vi "Sample-2.vi"() -> ()   [LabVIEW 2016]
uses:
  <vilib>/NI/Modbus Library/API/Wrapper/Create TCP Master.vi
  <vilib>/NI/Modbus Library/API/Wrapper/API Main.lvlib
panel:
  in  "Boolean 3":bool
  in  "stop":bool
  out "Tab Control":T1(tab)
  out "Boolean":bool
  out "SB-01-B-IAC 12":dbl
  out "SB-01-B-VAC 12":dbl
  out "SB-01-B-IAC 11":dbl
  out "SB-01-B-VAC 11":dbl
  out "SB-01-A-IAC 8":dbl
  out "SB-01-A-VAC 8":dbl
  out "SB-01-B-IAC 10":dbl
  out "SB-01-B-VAC 10":dbl
  out "SB-01-A-IAC 7":dbl
  out "SB-01-A-VAC 7":dbl
  out "SB-01-PAC 4":dbl
  out "SB-01-B-IAC 9":dbl
  out "SB-01-B-VAC 9":dbl
  out "SB-01-B-IAC 8":dbl
  out "SB-01-B-VAC 8":dbl
  out "SB-01-A-IAC 6":dbl
  out "SB-01-A-VAC 6":dbl
  out "SB-01-B-IAC 7":dbl
  out "SB-01-B-VAC 7":dbl
  out "SB-01-A-IAC 5":dbl
  out "SB-01-A-VAC 5":dbl
  out "SB-01-PAC 3":dbl
  out "SB-01-B-IAC 6":dbl
  out "SB-01-B-VAC 6":dbl
  out "SB-01-B-IAC 5":dbl
  out "SB-01-B-VAC 5":dbl
  out "SB-01-A-IAC 4":dbl
  out "SB-01-A-VAC 4":dbl
  out "SB-01-B-IAC 4":dbl
  out "SB-01-B-VAC 4":dbl
  out "SB-01-A-IAC 3":dbl
  out "SB-01-A-VAC 3":dbl
  out "SB-01-PAC 2":dbl
  out "SB-01-B-IAC 3":dbl
  out "SB-01-B-VAC 3":dbl
  out "SB-01-B-IAC 2":dbl
  out "SB-01-B-VAC 2":dbl
  out "SB-01-A-IAC 2":dbl
  out "SB-01-A-VAC 2":dbl
  out "SB-01-B-IAC":dbl
  out "SB-01-B-VAC":dbl
  out "SB-01-A-IAC":dbl
  out "SB-01-A-VAC":dbl
  out "SB-01-PAC":dbl
  out "PM-01-FREQ 2":dbl
  out "SI-M-FREQ 6":dbl
  out "SI-M-L3 6":dbl
  out "SI-M-L2 6":dbl
  out "SI-M-L1 6":dbl
  out "SI-M-PAC 6":dbl
  out "SI-M-FREQ 5":dbl
  out "SI-M-L3 5":dbl
  out "SI-M-L2 5":dbl
  out "SI-M-L1 5":dbl
  out "SI-M-PAC 5":dbl
  out "SI-M-FREQ 4":dbl
  out "SI-M-L3 4":dbl
  out "SI-M-L2 4":dbl
  out "SI-M-L1 4":dbl
  out "SI-M-PAC 4":dbl
  out "SI-M-FREQ 3":dbl
  out "SI-M-L3 3":dbl
  out "SI-M-L2 3":dbl
  out "SI-M-L1 3":dbl
  out "SI-M-PAC 3":dbl
  out "SI-M-FREQ 2":dbl
  out "SI-M-L3 2":dbl
  out "SI-M-L2 2":dbl
  out "SI-M-L1 2":dbl
  out "SI-M-PAC 2":dbl
  out "SI-M-FREQ":dbl
  out "SI-M-L3":dbl
  out "SI-M-L2":dbl
  out "SI-M-L1":dbl
  out "SI-M-PAC":dbl
  out "BANK-01-TEMP 2":dbl
  out "BANK-01-IDC 2":dbl
  out "BANK-01-VDC 2":dbl
  out "BANK-01-SOC 2":dbl
  out "BANK-01-TEMP":dbl
  out "BANK-01-IDC":dbl
  out "BANK-01-VDC":dbl
  out "BANK-01-SOC":dbl
  out "BANK-01-TEMP 4":dbl
  out "BANK-01-IDC 4":dbl
  out "BANK-01-VDC 4":dbl
  out "BANK-01-SOC 4":dbl
  out "BANK-01-TEMP 3":dbl
  out "BANK-01-IDC 3":dbl
  out "BANK-01-VDC 3":dbl
  out "BANK-01-SOC 3":dbl
  out "PM-01-FREQ":dbl
  out "PM-01-IAC":dbl
  out "PM-01-VAC":dbl
  out "PM-01-PAC":dbl
  out "Boolean 2":bool
  in  "SB-05-IPADDRESS 3":string caption="SB-01-IPADDRESS"
  in  "SB-05-PORT 3":string
  in  "SB-04-PORT 2":string
  in  "SB-04-IPADDRESS 2":string caption="SB-01-IPADDRESS"
  in  "SB-03-PORT 2":string
  in  "SB-03-IPADDRESS 2":string caption="SB-01-IPADDRESS"
  in  "SB-02-PORT 2":string
  in  "SB-02-IPADDRESS 2":string caption="SB-01-IPADDRESS"
  in  "SB-01-PORT 2":string
  in  "SB-01-IPADDRESS 2":string caption="SB-01-IPADDRESS"
  in  "SB-05-IPADDRESS 2":string caption="SB-01-IPADDRESS"
  in  "SB-05-PORT 2":string
  in  "INTERVAL":string(combo)
  in  "setting_save_mysql":bool
  in  "db_pwd":string caption="SB-01-IPADDRESS"
  in  "db_username":string caption="SB-01-IPADDRESS"
  in  "db_database":string caption="SB-01-IPADDRESS"
  in  "db_port":string caption="SB-01-IPADDRESS"
  in  "db_host":string caption="SB-01-IPADDRESS"
  in  "db_connection":string caption="SB-01-IPADDRESS"
  in  "setting_save":bool
  in  "SB-04-PORT":string
  in  "SB-04-IPADDRESS":string caption="SB-01-IPADDRESS"
  in  "SB-03-PORT":string
  in  "SB-03-IPADDRESS":string caption="SB-01-IPADDRESS"
  in  "SB-02-PORT":string
  in  "SB-02-IPADDRESS":string caption="SB-01-IPADDRESS"
  in  "SB-01-PORT":string
  in  "SB-01-IPADDRESS":string
  in  "SB-05-IPADDRESS":string caption="SB-01-IPADDRESS"
  in  "SB-05-PORT":string
  in  "Multicolumn Listbox":i32(listbox)
  in  "Path":path
  in  "DATE_END":timestamp format="%<%d/%m/%Y>T"
  in  "DATE_START":timestamp format="%<%d/%m/%Y>T"
  in  "DOWNLOAD":bool
  out "AC_VOLTAGE":cluster{dbl, dbl}[](graph)
  out "BATTERY_CURRENT":cluster{dbl, dbl}[](graph)
  out "SOC":cluster{dbl, dbl}[](graph)
  out "AC_POWER":cluster{dbl, dbl}[](graph)
  in  "Radio Buttons":T2(radio)
  # "RUMAH BUJAH ( 36.58 kWp )"
  # "STP-01"
  # "C.Vdc(V)"
  # "BANK-1"
  # "BANK-2"
  # "BANK-3"
  # "BANK-4"
  # "Pac (W)"
  # "C.Idc(A)"
  # "SOC (%)"
  # "SOC (%)"
  # "SOC (%)"
  # "SOC (%)"
  # "A.Vdc(V)"
  # "D.Vdc(V)"
  # "V_bat(V)"
  # "V_bat(V)"
  # "V_bat(V)"
  # "V_bat(V)"
  # "A.Idc(A)"
  # "D.Idc(A)"
  # "I_bat(A)"
  # "I_bat(A)"
  # "I_bat(A)"
  # "I_bat(A)"
  # "B.Vdc(V)"
  # "E.Vdc(V)"
  # "T_bat(°C)"
  # "T_bat(°C)"
  # "T_bat(°C)"
  # "T_bat(°C)"
  # "B.Idc(A)"
  # "E.Idc(A)"
  # "SI-M"
  # "SI-M"
  # "SI-01"
  # "SI-02"
  # "SI-01"
  # "SI-02"
  # "Pac (W)"
  # "Pac (W)"
  # "Pac (W)"
  # "Pac (W)"
  # "Pac (W)"
  # "Pac (W)"
  # "L1"
  # "L1"
  # "L1"
  # "L1"
  # "L1"
  # "L1"
  # "L2"
  # "L2"
  # "L2"
  # "L2"
  # "L2"
  # "L2"
  # "L3"
  # "L3"
  # "L3"
  # "L3"
  # "L3"
  # "L3"
  # "Fz(HZ)"
  # "Fz(HZ)"
  # "Fz(HZ)"
  # "Fz(HZ)"
  # "Fz(HZ)"
  # "Fz(HZ)"
  # "PM-01"
  # "Pac(W)"
  # "L1"
  # "L2"
  # "L3"
  # "fz(hz)"
  # "STP-04"
  # "C.Vdc(V)"
  # "Pac (W)"
  # "C.Idc(A)"
  # "A.Vdc(V)"
  # "D.Vdc(V)"
  # "A.Idc(A)"
  # "D.Idc(A)"
  # "B.Vdc(V)"
  # "E.Vdc(V)"
  # "B.Idc(A)"
  # "E.Idc(A)"
  # "STP-03"
  # "C.Vdc(V)"
  # "Pac (W)"
  # "C.Idc(A)"
  # "A.Vdc(V)"
  # "D.Vdc(V)"
  # "A.Idc(A)"
  # "D.Idc(A)"
  # "B.Vdc(V)"
  # "E.Vdc(V)"
  # "B.Idc(A)"
  # "E.Idc(A)"
  # "STP-02"
  # "C.Vdc(V)"
  # "Pac (W)"
  # "C.Idc(A)"
  # "A.Vdc(V)"
  # "D.Vdc(V)"
  # "A.Idc(A)"
  # "D.Idc(A)"
  # "B.Vdc(V)"
  # "E.Vdc(V)"
  # "B.Idc(A)"
  # "E.Idc(A)"
  # "SETTING"
  # "MODBUS TCP IP"
  # "MYSQL DATABASE"
  # "STP-01"
  # "SI-02"
  # "DB_CONNECTION :"
  # "IP ADDRESS"
  # "IP ADDRESS"
  # "DB_HOST :"
  # "PORT"
  # "PORT"
  # "DB_PORT  :"
  # "STP-02"
  # "SI-03"
  # "DB_DATABASE  :"
  # "IP ADDRESS"
  # "IP ADDRESS"
  # "DB_USERNAME  :"
  # "PORT"
  # "PORT"
  # "DB_PASSWORD  :"
  # "INTERVAL  :"
  # "STP-03"
  # "SI-04"
  # "IP ADDRESS"
  # "IP ADDRESS"
  # "PORT"
  # "PORT"
  # "STP-04"
  # "SI-05"
  # "IP ADDRESS"
  # "IP ADDRESS"
  # "PORT"
  # "PORT"
  # "SI-01"
  # "SI-06"
  # "IP ADDRESS"
  # "IP ADDRESS"
  # "PORT"
  # "PORT"
  # "DATA MANAGER"
  # "IP ADDRESS"
  # "PORT"
  # "ALERT LIST"
  # "DOWNLOAD DATA"
  # "FILE"
  # "DATE (START)"
  # "DATE (END)"
  # "CHART"
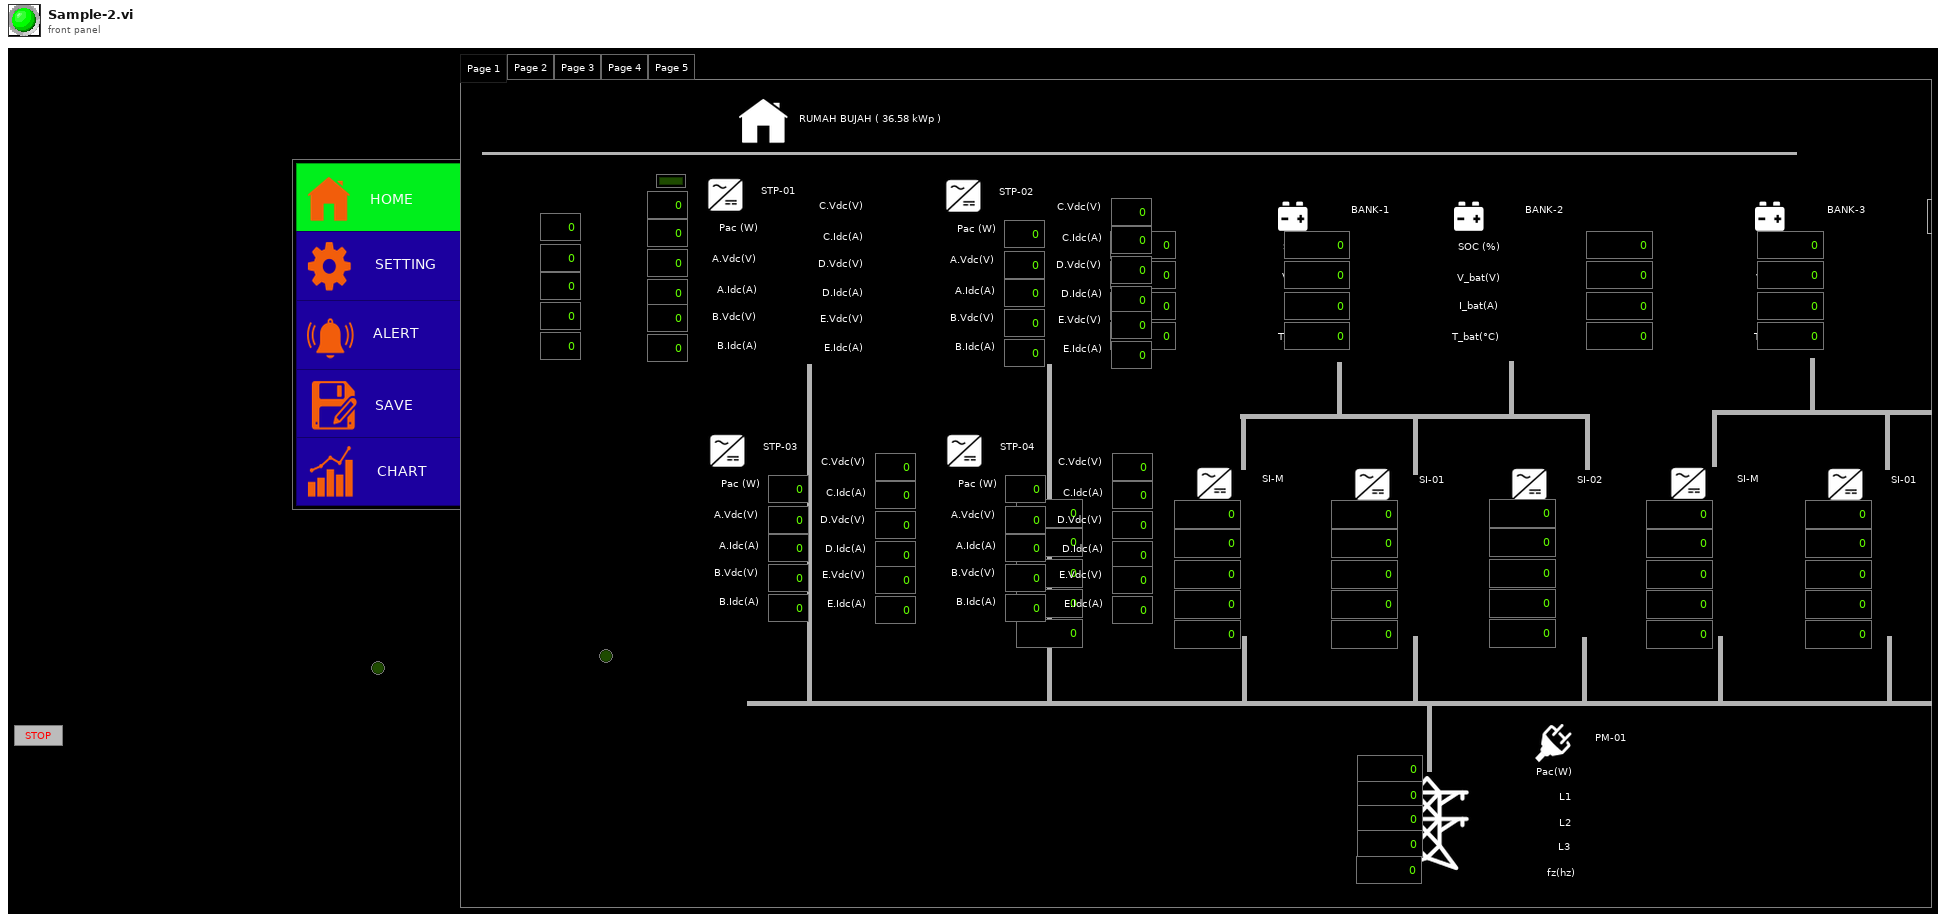
[diagram p1: front panel]
types:
  T1 = enum32{"Page 1", "Page 2", "Page 3", "Page 4", "Page 5"}
  T2 = enum32{"HOME", "SETTING", "ALERT", "SAVE", "CHART"}
  T3 = enum16{"open", "replace", "create", "open or create", "replace or create", "replace or create with confirmation"}
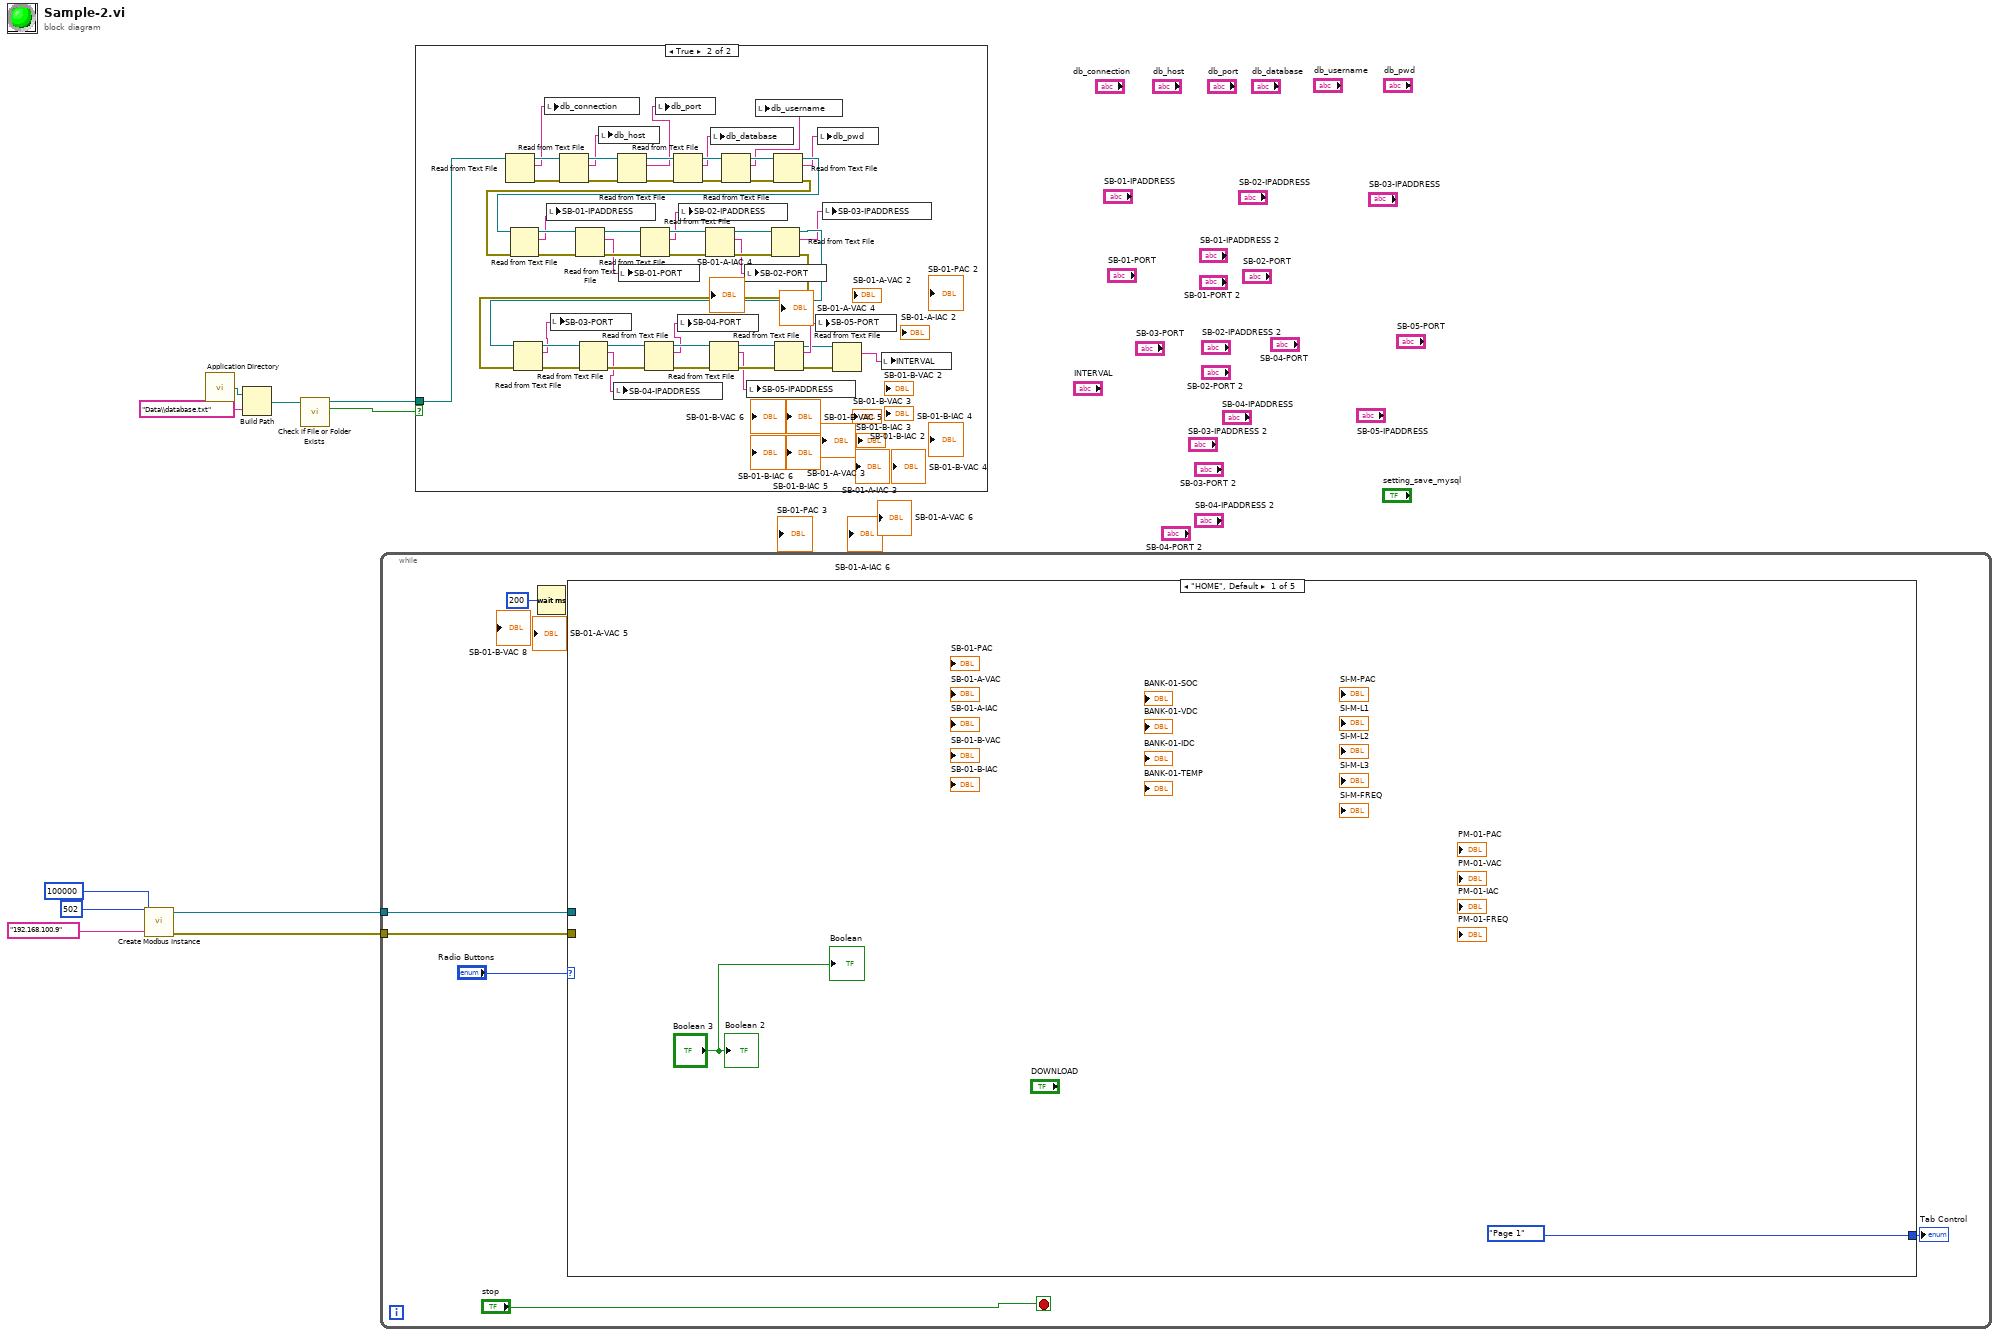
[diagram p0: block diagram]
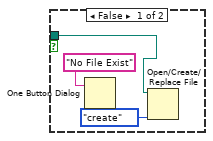
[diagram p2: hidden frame]
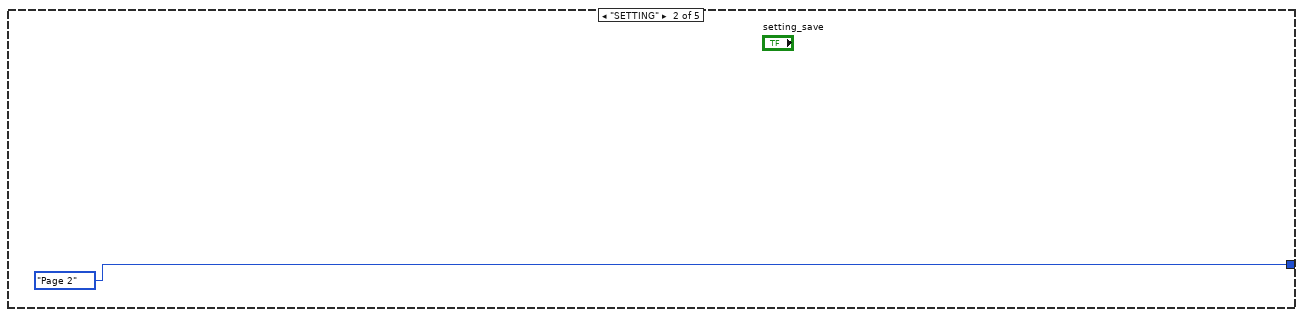
[diagram p3: hidden frame]
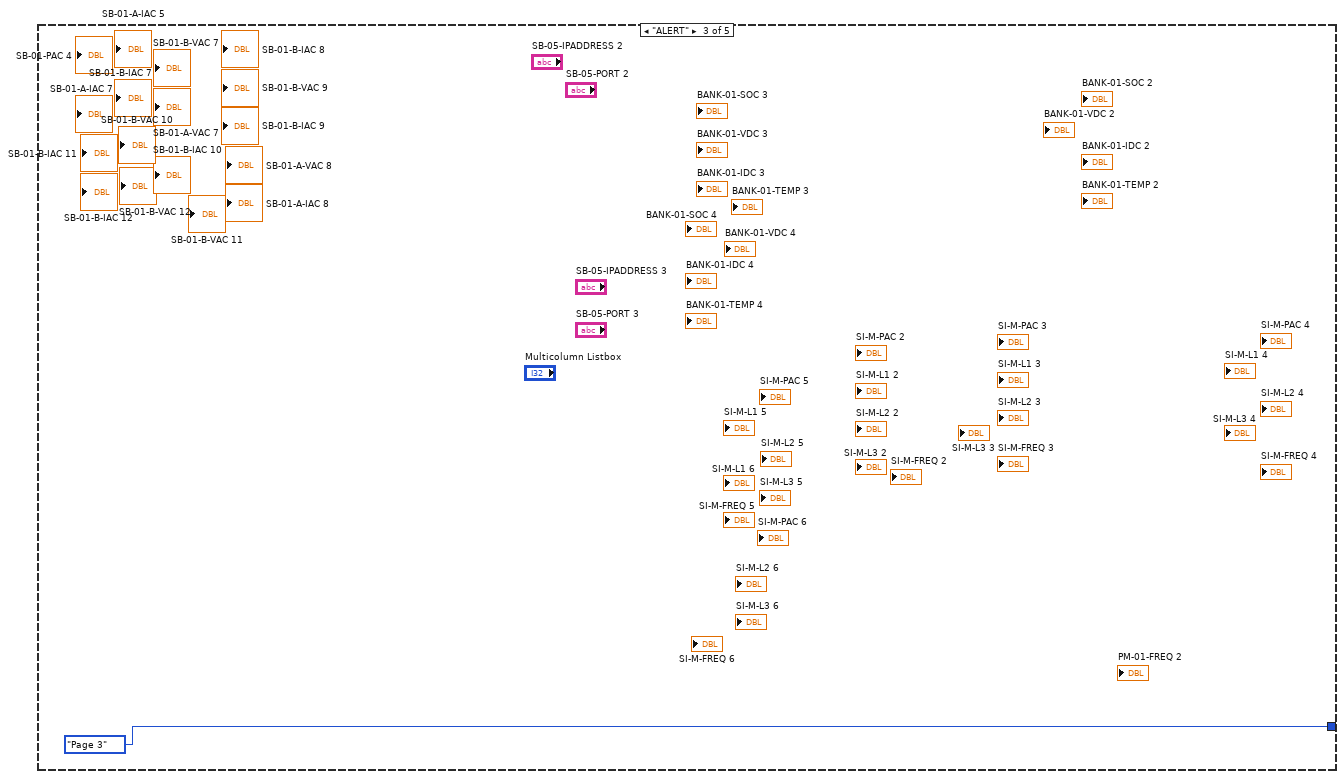
[diagram p4: hidden frame]
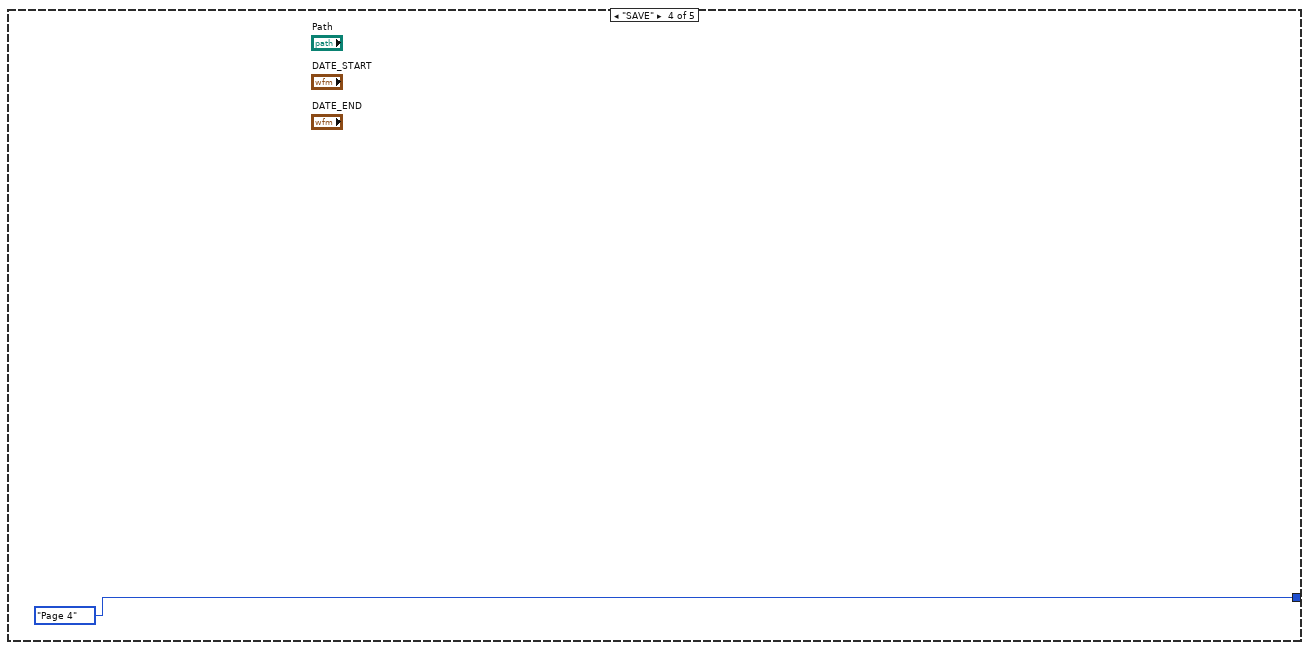
[diagram p5: hidden frame]
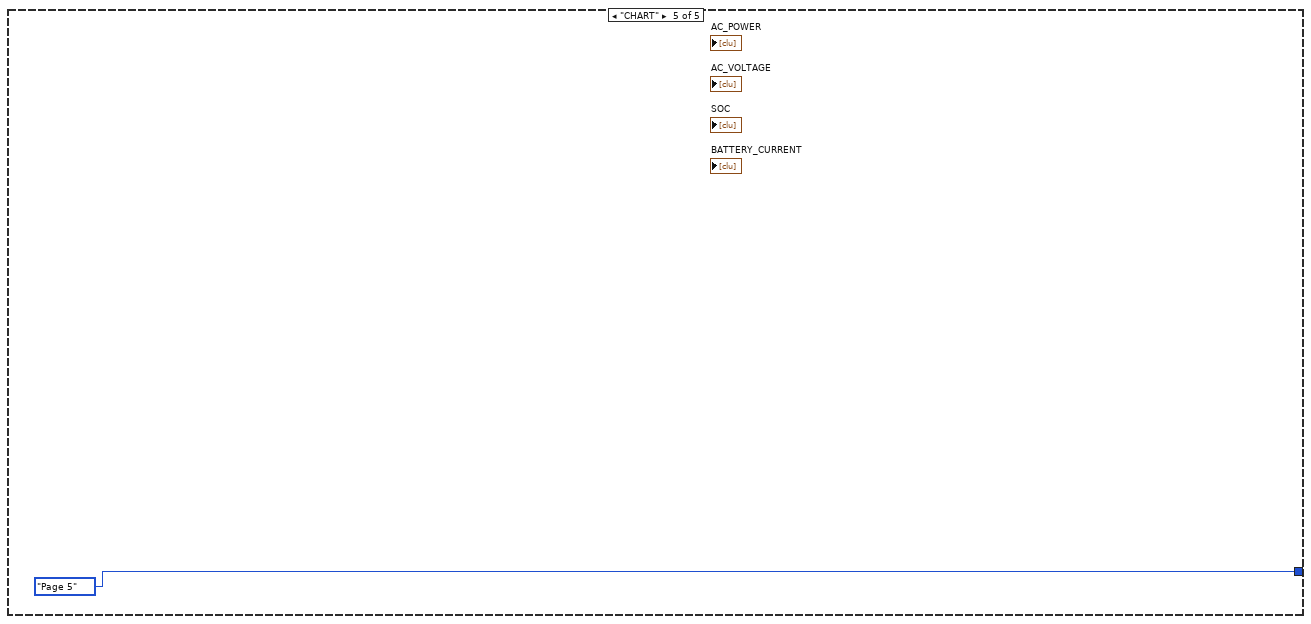
[diagram p6: hidden frame]
diagram:
  n1 = call-poly <vilib>:"Create Modbus Instance.vi"("connect timeout ms"=100000, "port (502)"=u16 502, "address"="192.168.100.9") -> ("error out"=w6:errorcluster, "TCP master instance"=w7:refnum<class "Modbus Master.lvclass">)  [unwired: 7 in]
  n2 = call <vilib>:"Application Directory.vi"() -> ("Application Directory"=w3:path)
  n3 = Build Path(base path=w3, name or relative path="Data\\database.txt") -> (appended path=w5:path)
  n4 = call <vilib>:"Check if File or Folder Exists.vi"("path"=w5) -> ("file or folder exists?"=w1:bool, "dup path"=w2:path)  [unwired: 8 in, 1 out]
  n5 = while {
    tunnel: w7 -> [w14]
    tunnel: w6 -> [w13]
    stop <- "stop" stop-if-true
    n6 = Wait (ms)(milliseconds to wait=u32 200) -> ()  [unwired: 1 out]
    n7 = case shown="\"HOME\", Default" "Radio Buttons" {
      tunnel: w14 -> [_ _ _ _ _]
      tunnel: w13 -> [_ _ _ _ _]
      tunnel: [T1."Page 1" ("Tab Control") T1."Page 2" ("Tab Control") T1."Page 3" ("Tab Control") T1."Page 4" ("Tab Control") T1."Page 5" ("Tab Control")] -> w11
      frame "HOME", Default {
        "Boolean 2" <- "Boolean 3"
        "Boolean" <- "Boolean 3"
      }
      frame "SETTING" {
      }
      frame "ALERT" {
      }
      frame "SAVE" {
      }
      frame "CHART" {
      }
    }
    "Tab Control" <- w11
  }
  n8 = case shown="True" w1 {
    tunnel: w2 -> [w24 w75]
    frame False {
      n9 = One Button Dialog(message="No File Exist") -> ()  [unwired: 1 in, 1 out]
      n10 = Open/Create/Replace File(file path (use dialog)=w24, operation (0:open)=T3."create") -> ()  [unwired: 4 in, 3 out]
    }
    frame True {
      n11 = Read from Text File(file (use dialog)=w75) -> (refnum out=w74:refnum<file>, text=w44:string, error out=w70:errorcluster)  [unwired: 3 in, 1 out]
      n12 = local write "db_connection"(w44) -> ()
      n13 = Read from Text File(file (use dialog)=w74, error in=w70) -> (refnum out=w73:refnum<file>, text=w43:string, error out=w69:errorcluster)  [unwired: 2 in, 1 out]
      n14 = local write "db_host"(w43) -> ()
      n15 = Read from Text File(file (use dialog)=w73, error in=w69) -> (refnum out=w72:refnum<file>, text=w42:string, error out=w68:errorcluster)  [unwired: 2 in, 1 out]
      n16 = local write "db_port"(w42) -> ()
      n17 = Read from Text File(file (use dialog)=w72, error in=w68) -> (refnum out=w71:refnum<file>, text=w41:string, error out=w67:errorcluster)  [unwired: 2 in, 1 out]
      n18 = local write "db_database"(w41) -> ()
      n19 = Read from Text File(file (use dialog)=w71, error in=w67) -> (refnum out=w66:refnum<file>, text=w40:string, error out=w65:errorcluster)  [unwired: 2 in, 1 out]
      n20 = local write "db_username"(w40) -> ()
      n21 = Read from Text File(file (use dialog)=w66, error in=w65) -> (refnum out=w63:refnum<file>, text=w39:string, error out=w64:errorcluster)  [unwired: 2 in, 1 out]
      n22 = Read from Text File(file (use dialog)=w63, error in=w64) -> (refnum out=w62:refnum<file>, text=w38:string, error out=w50:errorcluster)  [unwired: 2 in, 1 out]
      n23 = local write "SB-01-IPADDRESS"(w38) -> ()
      n24 = Read from Text File(file (use dialog)=w62, error in=w50) -> (refnum out=w61:refnum<file>, text=w37:string, error out=w49:errorcluster)  [unwired: 2 in, 1 out]
      n25 = local write "SB-01-PORT"(w37) -> ()
      n26 = Read from Text File(file (use dialog)=w61, error in=w49) -> (refnum out=w60:refnum<file>, text=w36:string, error out=w48:errorcluster)  [unwired: 2 in, 1 out]
      n27 = local write "SB-02-IPADDRESS"(w36) -> ()
      n28 = Read from Text File(file (use dialog)=w60, error in=w48) -> (refnum out=w59:refnum<file>, text=w35:string, error out=w47:errorcluster)  [unwired: 2 in, 1 out]
      n29 = local write "SB-02-PORT"(w35) -> ()
      n30 = Read from Text File(file (use dialog)=w59, error in=w47) -> (refnum out=w45:refnum<file>, text=w34:string, error out=w46:errorcluster)  [unwired: 2 in, 1 out]
      n31 = Read from Text File(file (use dialog)=w45, error in=w46) -> (refnum out=w58:refnum<file>, text=w32:string, error out=w54:errorcluster)  [unwired: 2 in, 1 out]
      n32 = local write "SB-03-PORT"(w32) -> ()
      n33 = Read from Text File(file (use dialog)=w58, error in=w54) -> (refnum out=w57:refnum<file>, text=w33:string, error out=w53:errorcluster)  [unwired: 2 in, 1 out]
      n34 = local write "SB-04-IPADDRESS"(w33) -> ()
      n35 = Read from Text File(file (use dialog)=w57, error in=w53) -> (refnum out=w56:refnum<file>, text=w31:string, error out=w52:errorcluster)  [unwired: 2 in, 1 out]
      n36 = local write "SB-04-PORT"(w31) -> ()
      n37 = Read from Text File(file (use dialog)=w56, error in=w52) -> (refnum out=w55:refnum<file>, text=w30:string, error out=w51:errorcluster)  [unwired: 2 in, 1 out]
      n38 = local write "SB-05-IPADDRESS"(w30) -> ()
      n39 = Read from Text File(file (use dialog)=w55, error in=w51) -> (refnum out=w28:refnum<file>, text=w29:string, error out=w27:errorcluster)  [unwired: 2 in, 1 out]
      n40 = local write "SB-05-PORT"(w29) -> ()
      n41 = local write "db_pwd"(w39) -> ()
      n42 = local write "SB-03-IPADDRESS"(w34) -> ()
      n43 = Read from Text File(file (use dialog)=w28, error in=w27) -> (text=w26:string)  [unwired: 2 in, 3 out]
      n44 = local write "INTERVAL"(w26) -> ()
    }
  }
